vi "IncorrectResponse.vi"(8 "error in (no error)":errorcluster, 11 "TrialBasedExperiment in":refnum<class "WhiteNoiseOrientationDetection.lvclass">) -> (0 "error out":errorcluster, 3 "TrialBasedExperiment out":refnum<class "WhiteNoiseOrientationDetection.lvclass">)   [LabVIEW 2012, in "WhiteNoiseOrientationDetection.lvclass"]
uses:
  WhiteNoiseOrientationDetection.lvclass
  Trial Based Experiment Statechart/MatlabExperiment/MatlabExperiment.lvclass
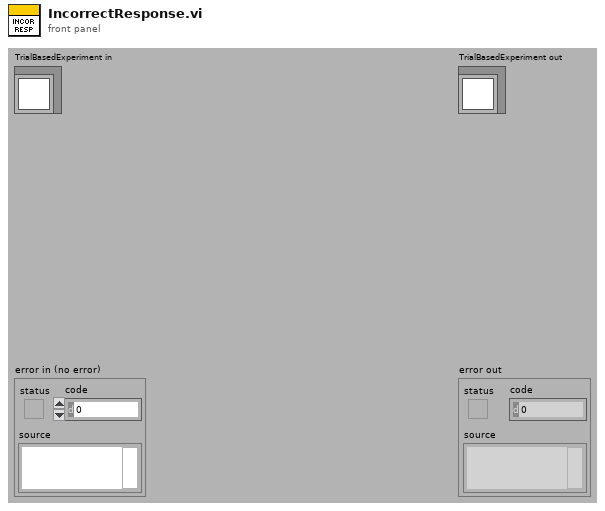
[diagram p1: front panel]
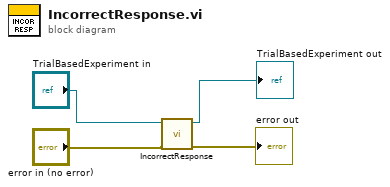
[diagram p0: block diagram]
diagram:
  n1 = call-parent "IncorrectResponse.vi"("error in (no error)"="error in (no error)", "TrialBasedExperiment in"="TrialBasedExperiment in") -> ("error out"=→"error out":errorcluster, "TrialBasedExperiment out"=→"TrialBasedExperiment out":refnum<class "WhiteNoiseOrientationDetection.lvclass">)  [unwired: 8 in]
